vi "TB-Save Setup Log.vi"(0 "State":T3, 1 "VI ref":refnum<vi>, 5 "Exposure parameters":T1={"Low cutoff (kHz)"=0.0, "High cutoff (kHz)"=0.0, "Duration (min)"=0.0, "dB SPL"=0.0, "Waveform"=enum."OFF", "WAVfile"=path "", "refWav"=path "", "use mic correction"=FALSE, "micCorrFile"=path "", "Pistonphone Level (dB SPL)"=0.0, "Sampling rate (Hz)"=0.0, "Buffer length (s)"=0.0, "Stream mic"=FALSE, "Fine adjust"={"Max"=0.0, "Min"=0.0}, "Mic gain"=0.0, "atten"=0.0, "resol (Hz)"=0.0, "navgs"=0, "Allow Slack"=FALSE, "max starts"=0, "Freq (kHz)"=8.0, "Tma (s)"=0.0, "Streamed"=[], "Drive"=""}, 12 "Fine Control":dbl) -> (8 "date/time string":string, 15 "error out":errorcluster)   [LabVIEW 2020]
uses:
  Typedefs/TB-Runtime state.ctl
  <vilib>/sound2/lvsound2.llb/Sound File Refnum.ctl
  Typedefs/TB-Setup Log.ctl
  Typedefs/TB-Parameters.ctl
  epl-vi-lib/Signal Synthesis VIs/Controls/Waveform XCtl/Waveform Enum.ctl
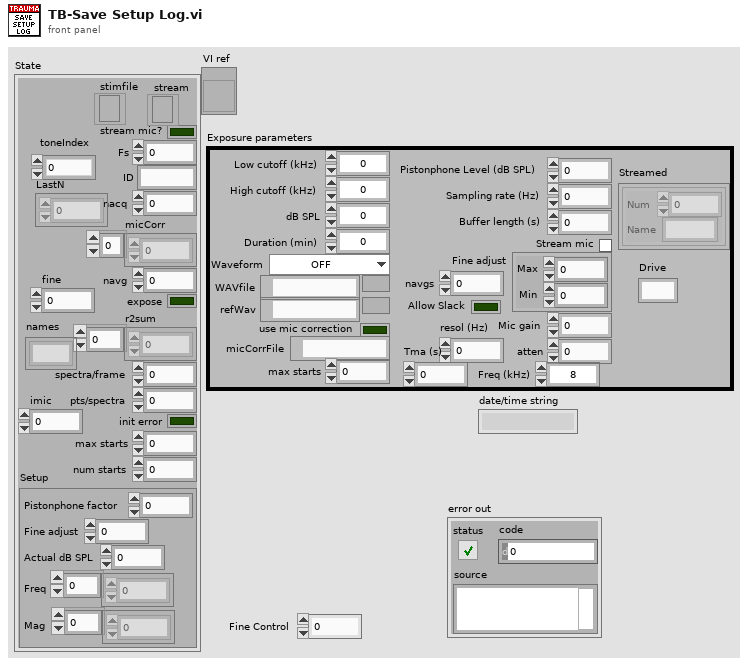
[diagram p1: front panel]
types:
  T1 = typedef "TB-Parameters.ctl" = cluster{"Low cutoff (kHz)":dbl, "High cutoff (kHz)":dbl, "Duration (min)":dbl, "dB SPL":dbl, "Waveform":T2, "WAVfile":path, "refWav":path, "use mic correction":bool, "micCorrFile":path, "Pistonphone Level (dB SPL)":dbl, "Sampling rate (Hz)":dbl, "Buffer length (s)":dbl, "Stream mic":bool, "Fine adjust":cluster{"Max":dbl, "Min":dbl}, "Mic gain":dbl, "atten":dbl, "resol (Hz)":dbl, "navgs":i32, "Allow Slack":bool, "max starts":i32, "Freq (kHz)":dbl, "Tma (s)":dbl, "Streamed":cluster{"Num":i32, "Name":string}[], "Drive":string}
  T2 = typedef "Waveform Enum.ctl" = enum16{"OFF", "Tone", "Noise", "Pulse Train", "File", "FM Sweep", "Chirp Train", "Complex Tone", "FM Tone", "Moving Ripple"}
  T3 = typedef "TB-Runtime state.ctl" = cluster{"stimfile":T4, "stream mic?":bool, "Fs":dbl, "ID":string, "micCorr":dbl[], "navg":i32, "r2sum":dbl[], "expose":bool, "spectra/frame":i32, "pts/spectra":i32, "nacq":i32, "init error":bool, "max starts":i32, "num starts":i32, "Setup":T5, "toneIndex":i32, "LastN":dbl[], "fine":dbl, "imic":i32, "stream":refnum<file>, "names":string[]}
  T4 = typedef "Sound File Refnum.ctl" = refnum<file>
  T5 = typedef "TB-Setup Log.ctl" = cluster{"Pistonphone factor":dbl, "Fine adjust":dbl, "Actual dB SPL":dbl, "Freq":dbl[], "Mag":dbl[]}
  T6 = typedef "imagedata.ctl" = cluster{"image type":i32, "image depth":i32, "image":u8[], "mask":u8[], "colors":u32[], "Rectangle":cluster{"left":i16, "top":i16, "right":i16, "bottom":i16}}
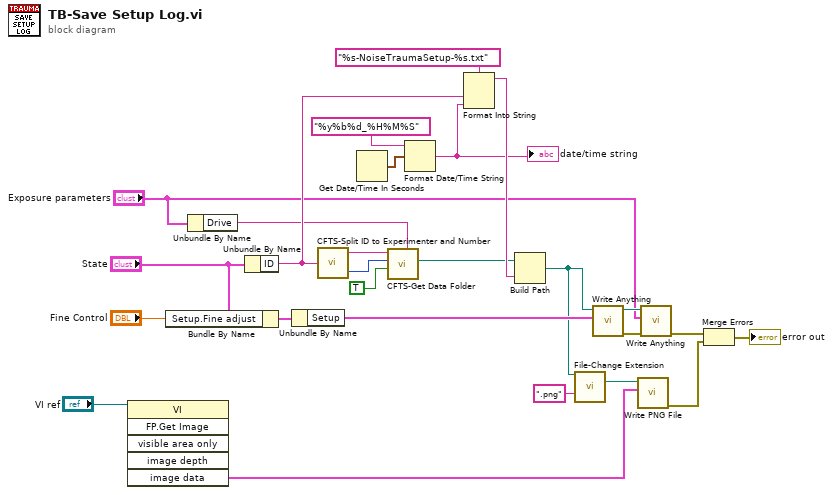
[diagram p0: block diagram]
diagram:
  n1 = invoke class="VI" method="FP.Get Image"(reference="VI ref") -> ("image data"=w3:T6)  [unwired: 5 in, 5 out]
  n2 = Bundle By Name(cluster="State", "Setup.Fine adjust"="Fine Control") -> (w15:T3)
  n3 = Unbundle By Name("Exposure parameters") -> ("Drive"=w1:string)
  n4 = Unbundle By Name("State") -> ("ID"=w19:string)
  n5 = Unbundle By Name(w15) -> ("Setup"=w14:T5)
  n6 = call "CFTS-Split ID to Experimenter and Number.vi"("ID"=w19) -> ("Experimenter"=w25:string, "Number"=w26:i32)
  n7 = Get Date/Time In Seconds() -> (seconds since 1Jan1904=w22:timestamp)
  n8 = call "CFTS-Get Data Folder.vi"("Drive"=w1, "create?"=TRUE, "Number"=w26, "Experimenter"=w25) -> ("Data folder"=w9:path)  [unwired: 6 in, 1 out]
  n9 = Format Date/Time String(time format string (%c)="%y%b%d_%H%M%S", seconds (now)=w22) -> (date/time string=w20:string)  [unwired: 1 in]
  "date/time string" <- w20
  n10 = Format Into String(format string="%s-NoiseTraumaSetup-%s.txt", w19, w20) -> (resulting string=w23:string)  [unwired: 2 in, 1 out]
  n11 = Build Path(base path=w9, name or relative path=w23) -> (appended path=w8:path)
  n12 = call "File-Change Extension.vi"("Path"=w8, "new extension"=".png") -> ("new path"=w6:path)  [unwired: 13 in]
  n13 = call "Write Anything.vi"("Anything"=w14, "Path (dialog)"=w8) -> ("Error Out"=w12:errorcluster, "Path out"=w13:path)  [unwired: 8 in]
  n14 = call <vilib>:"Write PNG File.vi"("image data"=w3, "path to PNG file"=w6) -> ("error out"=w4:errorcluster)  [unwired: 8 in, 1 out]
  n15 = call "Write Anything.vi"("Error In"=w12, "Anything"="Exposure parameters", "Path (dialog)"=w13) -> ("Error Out"=w11:errorcluster)  [unwired: 7 in, 1 out]
  n16 = Merge Errors(w11, w4) -> (→"error out":errorcluster)
